vi "FB Server.vi"(0 "C2O":dbl[][](array[numeric])) -> (7 "Fx                     Fy                     Fz                    Mx                   My                    Mz":dbl[](array[numeric])=[0.39367133033328505, 0.12640519158271346, -0.035168369141984894, 0.07356448847559971, 0.08928756090020755, 0.03408632169703757])   [LabVIEW 2017]
uses:
  <vilib>/Analysis/baseanly.llb/Mean (DBL).vi
  <vilib>/Analysis/baseanly.llb/A x Vector.vi
  <vilib>/Utility/file.llb/Write To Spreadsheet File (DBL).vi
  <vilib>/Utility/file.llb/Read From Spreadsheet File (DBL).vi
  <vilib>/Analysis/NI_AALBase.lvlib
panel:
  in  "Sampling Period":dbl=30.0
  in  "Sampling Freq.":dbl=500.0
  in  "x":bool
  in  "stop":bool
  out "Waveform Chart":dynamicdata(graph)=[{"t0"=timestamp(3625740071.8186145 s since 1904-01-01), "dt"=0.002, "Y"=[1.4132434446437658, 1.4869062871436736, 1.4652020568354351, 1.4342899711432204, 1.515516408827019], "attributes"=variant("NI_ChannelName"=variant(string "Voltage_0"), "NI_UnitDescription"=variant(string "Volts"))}, {"t0"=timestamp(3625740071.8186283 s since 1904-01-01), "dt"=0.002, "Y"=[0.4493782119596065, 0.441156910799936, 0.42537201251587176, 0.4112313744050537, 0.41221793055431444], "attributes"=variant("NI_ChannelName"=variant(string "Voltage_1"), "NI_UnitDescription"=variant(string "Volts"))}, {"t0"=timestamp(3625740071.818642 s since 1904-01-01), "dt"=0.002, "Y"=[0.1241435215364698, 0.13861301307479987, 0.18070607894651378, 0.13466678811720997, 0.12841859858966923], "attributes"=variant("NI_ChannelName"=variant(string "Voltage_2"), "NI_UnitDescription"=variant(string "Volts"))}, {"t0"=timestamp(3625740071.8186564 s since 1904-01-01), "dt"=0.002, "Y"=[4.929329220143692, 4.876055168157049, 4.92110791573665, 4.952020020475538, 4.8872361419192885], "attributes"=variant("NI_ChannelName"=variant(string "Voltage_3"), "NI_UnitDescription"=variant(string "Volts"))}, {"t0"=timestamp(3625740071.8186703 s since 1904-01-01), "dt"=0.002, "Y"=[1.7019754755920375, 1.6973715480570852, 1.6858617292118738, 1.741437711535304, 1.7019754755920375], "attributes"=variant("NI_ChannelName"=variant(string "Voltage_4"), "NI_UnitDescription"=variant(string "Volts"))}, {"t0"=timestamp(3625740071.8186846 s since 1904-01-01), "dt"=0.002, "Y"=[-1.6523161496933905, -1.626994516567589, -1.6023305886073516, -1.6164712405886696, -1.6292964831977657], "attributes"=variant("NI_ChannelName"=variant(string "Voltage_5"), "NI_UnitDescription"=variant(string "Volts"))}]
  out "L2                   S                  D2                  L1                  L3                  D1":dbl[](array[numeric])=[1.4630316337186229, 0.42787128804695646, 0.14130960005293253, 1.7057243879976673, 4.913149693286444, -1.6254817957309533]
  out "Amber Check":bool[](array[boolean])
  out "Amber Check Fail":bool
  out "OMFG Check":bool[](array[boolean])
  out "OMFG Check Fail":bool
  out "Mean Convergence":dbl(graph)=0.08995560655426219
  in  "Blank Button":bool
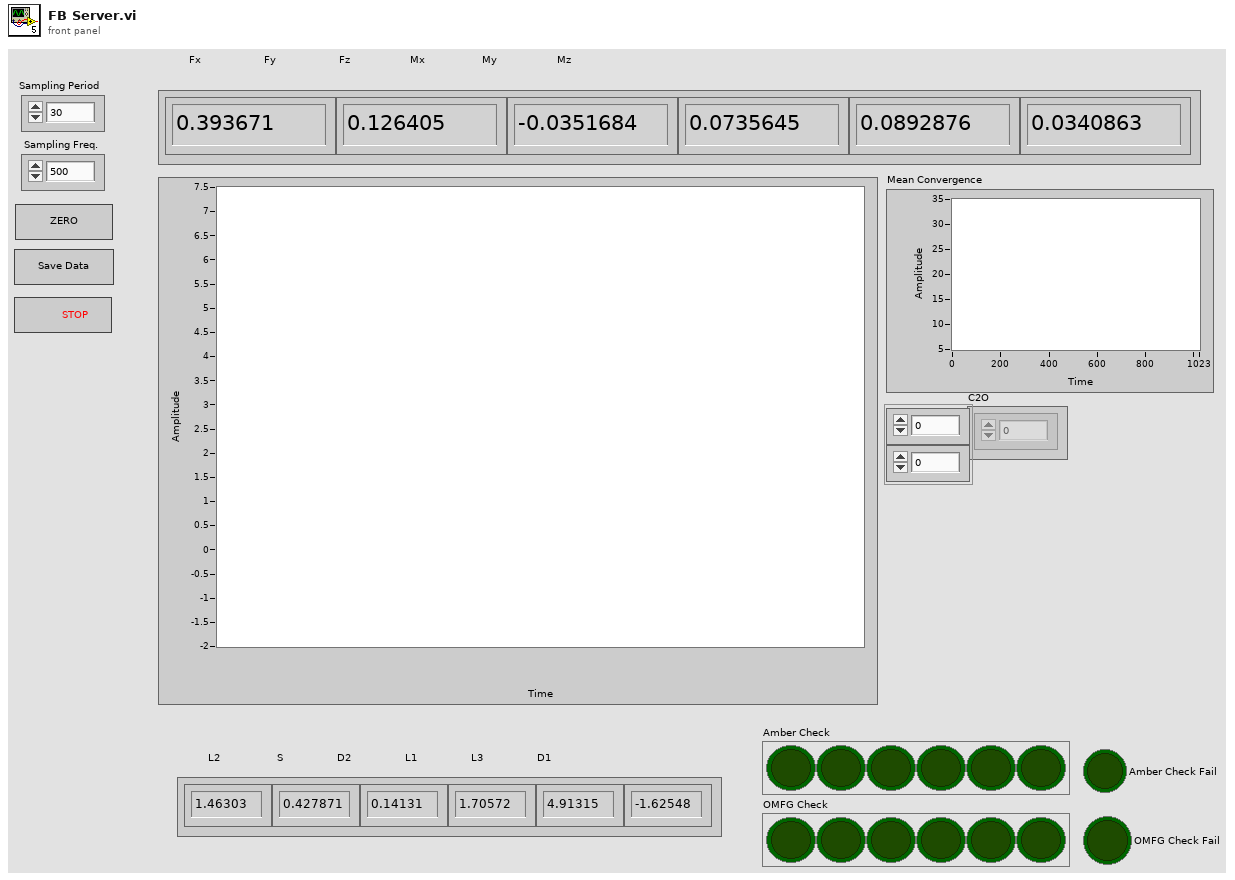
[diagram p1: front panel]
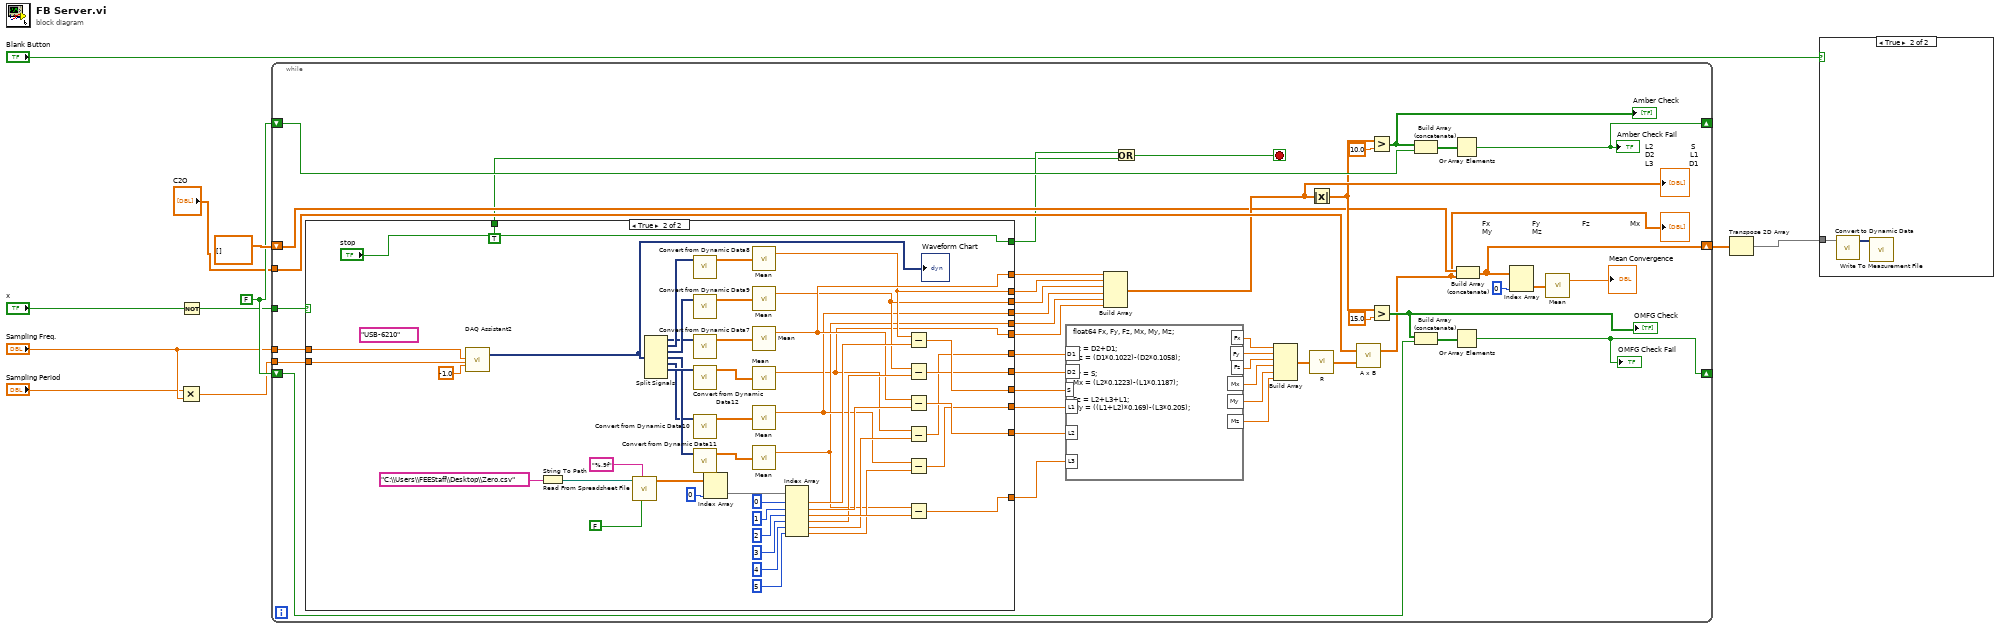
[diagram p0: block diagram]
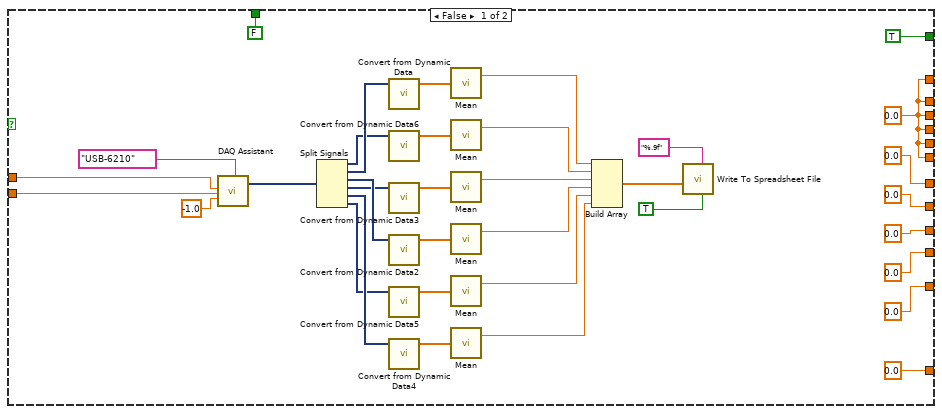
[diagram p3: hidden frame]
diagram:
  w9 = FALSE
  n1 = Multiply(x="Sampling Period", y="Sampling Freq.") -> (x*y=w7:dbl)
  n2 = Not(x="x") -> (.not. x?=w3:bool)
  n3 = while {
    tunnel: w3 -> [w56]
    tunnel: "Sampling Freq." -> [w55]
    tunnel: w7 -> [w54]
    tunnel: "C2O" -> [w53]
    shift-right: [w17] -> _
    shift-left: w9 -> [w30]
    shift-right: [w18] -> _
    shift-left: w9 -> [w25]
    shift-right: [w19] -> w11
    shift-left: dbl[][] [] -> [w20]
    stop <- w14 stop-if-true
    n4 = case shown="True" w56 {
      tunnel: [0.0 w107] -> w46
      tunnel: [0.0 w106] -> w45
      tunnel: [0.0 w125] -> w49
      tunnel: [0.0 w124] -> w48
      tunnel: [0.0 w126] -> w47
      tunnel: [0.0 w127] -> w50
      tunnel: w55 -> [w91 w140]
      tunnel: w54 -> [w90 w139]
      tunnel: [TRUE ("stop") "stop"] -> w15
      tunnel: [w58 w98] -> w38
      tunnel: [w58 w97] -> w37
      tunnel: [w58 w96] -> w36
      tunnel: [w58 w95] -> w35
      tunnel: [w58 w94] -> w34
      tunnel: [w58 w93] -> w33
      tunnel: [FALSE ("stopped") TRUE ("stopped")] -> w12
      frame False {
        w58 = 0.0
        n5 = call "DAQ Assistant"("rate"=w91, "number of samples"=w90, "timeout (s)"=-1.0, "device name"=tag "USB-6210") -> ("data"=w77:dynamicdata)  [unwired: 13 in, 2 out]
        n6 = Split Signals(w77) -> (w65:dynamicdata, w76:dynamicdata, w74:dynamicdata, w72:dynamicdata, w70:dynamicdata, w68:dynamicdata)  [unwired: 6 in]
        n7 = call "Convert from Dynamic Data"("Dynamic Data Type"=w76) -> ("Array"=w75:dbl[])  [unwired: 3 in]
        n8 = call "Convert from Dynamic Data6"("Dynamic Data Type"=w65) -> ("Array"=w61:dbl[])  [unwired: 3 in]
        n9 = call "Convert from Dynamic Data3"("Dynamic Data Type"=w72) -> ("Array"=w71:dbl[])  [unwired: 3 in]
        n10 = call "Convert from Dynamic Data2"("Dynamic Data Type"=w74) -> ("Array"=w73:dbl[])  [unwired: 3 in]
        n11 = call "Convert from Dynamic Data5"("Dynamic Data Type"=w68) -> ("Array"=w67:dbl[])  [unwired: 3 in]
        n12 = call "Convert from Dynamic Data4"("Dynamic Data Type"=w70) -> ("Array"=w69:dbl[])  [unwired: 3 in]
        n13 = call-poly <vilib>:"Mean.vi"("X"=w75) -> ("mean"=w82:dbl)  [unwired: 1 out]
        n14 = call-poly <vilib>:"Mean.vi"("X"=w61) -> ("mean"=w79:dbl)  [unwired: 1 out]
        n15 = call-poly <vilib>:"Mean.vi"("X"=w71) -> ("mean"=w62:dbl)  [unwired: 1 out]
        n16 = call-poly <vilib>:"Mean.vi"("X"=w73) -> ("mean"=w81:dbl)  [unwired: 1 out]
        n17 = call-poly <vilib>:"Mean.vi"("X"=w67) -> ("mean"=w80:dbl)  [unwired: 1 out]
        n18 = call-poly <vilib>:"Mean.vi"("X"=w69) -> ("mean"=w60:dbl)  [unwired: 1 out]
        n19 = Build Array(w82, w79, w62, w81, w80, w60) -> (w78:dbl[])
        n20 = call-poly <vilib>:"Write To Spreadsheet File.vi"("transpose? (no:F)"=TRUE, "format (%.3f)"="%.9f", "1D data"=w78) -> ()  [unwired: 5 in, 1 out]
      }
      frame True {
        (unwired) tag "USB-6210" ("device name")
        n21 = call "DAQ Assistant2"("rate"=w140, "number of samples"=w139, "timeout (s)"=-1.0) -> ("data"=w99:dynamicdata)  [unwired: 14 in, 2 out]
        "Waveform Chart" <- w99
        n22 = String To Path(string="C:\\Users\\FEEStaff\\Desktop\\Zero.csv" ("format (%.3f)")) -> (path=w108:path)
        n23 = call-poly <vilib>:"Read From Spreadsheet File.vi"("transpose (no:F)"=FALSE, "format (%.3f)"="%.9f", "file path (dialog if empty)"=w108) -> ("all rows"=w130:dbl[][])  [unwired: 4 in, 4 out]
        n24 = Split Signals(w99) -> (w115:dynamicdata, w121:dynamicdata, w119:dynamicdata, w102:dynamicdata, w101:dynamicdata, w116:dynamicdata)  [unwired: 7 in, 1 out]
        n25 = call "Convert from Dynamic Data8"("Dynamic Data Type"=w121) -> ("Array"=w120:dbl[])  [unwired: 3 in]
        n26 = call "Convert from Dynamic Data9"("Dynamic Data Type"=w119) -> ("Array"=w104:dbl[])  [unwired: 3 in]
        n27 = call "Convert from Dynamic Data7"("Dynamic Data Type"=w115) -> ("Array"=w122:dbl[])  [unwired: 3 in]
        n28 = call "Convert from Dynamic Data12"("Dynamic Data Type"=w116) -> ("Array"=w105:dbl[])  [unwired: 3 in]
        n29 = call "Convert from Dynamic Data10"("Dynamic Data Type"=w101) -> ("Array"=w118:dbl[])  [unwired: 3 in]
        n30 = call "Convert from Dynamic Data11"("Dynamic Data Type"=w102) -> ("Array"=w117:dbl[])  [unwired: 3 in]
        n31 = Index Array(array=w130, index (col)=0 ("disabled index (col)")) -> (element=w128:dbl[])  [unwired: 1 in]
        n32 = call-poly <vilib>:"Mean.vi"("X"=w120) -> ("mean"=w97:dbl)  [unwired: 1 out]
        n33 = call-poly <vilib>:"Mean.vi"("X"=w104) -> ("mean"=w96:dbl)  [unwired: 1 out]
        n34 = call-poly <vilib>:"Mean.vi"("X"=w122) -> ("mean"=w98:dbl)  [unwired: 1 out]
        n35 = call-poly <vilib>:"Mean.vi"("X"=w105) -> ("mean"=w93:dbl)  [unwired: 1 out]
        n36 = call-poly <vilib>:"Mean.vi"("X"=w118) -> ("mean"=w95:dbl)  [unwired: 1 out]
        n37 = call-poly <vilib>:"Mean.vi"("X"=w117) -> ("mean"=w94:dbl)  [unwired: 1 out]
        n38 = Index Array(array=w128, index #1=0 ("index (row)"), index #2=1 ("index (row)"), index #3=2 ("index (row)"), index #4=3 ("index (row)"), index #5=4 ("index (row)"), index #6=5 ("index (row)")) -> (element #1=w114:dbl, element #2=w113:dbl, element #3=w112:dbl, element #4=w111:dbl, element #5=w110:dbl, element #6=w103:dbl)
        n39 = Subtract(x=w97, y=w114) -> (x-y=w127:dbl)
        n40 = Subtract(x=w96, y=w111) -> (x-y=w107:dbl)
        n41 = Subtract(x=w98, y=w113) -> (x-y=w125:dbl)
        n42 = Subtract(x=w93, y=w110) -> (x-y=w106:dbl)
        n43 = Subtract(x=w95, y=w103) -> (x-y=w124:dbl)
        n44 = Subtract(x=w94, y=w112) -> (x-y=w126:dbl)
      }
    }
    n45 = formula code="float64 Fx, Fy, Fz, Mx, My, Mz;\n\nFx = D2+D1;\nMz = (D1*0.1022)-(D2*0.1058);\n\nFy = S;\nMx = (L2*0.1223)-(L1*0.1187);\n\nFz = L2+L3+L1;\nMy = ((L1+L2)*0.169)-(L3*0.205);"("D1"=w45, "D2"=w46, "S"=w50, "L1"=w48, "L2"=w49, "L3"=w47) -> ("Fx"=w44:dbl, "Fy"=w43:dbl, "Fz"=w42:dbl, "Mx"=w41:dbl, "My"=w40:dbl, "Mz"=w39:dbl)
    n46 = Build Array(w38, w37, w36, w35, w34, w33) -> (w32:dbl[])
    "L2                   S                  D2                  L1                  L3                  D1" <- w32
    n47 = Or(x=w15, y=w12) -> (x .or. y?=w14:bool)
    n48 = Build Array(w44, w43, w42, w41, w40, w39) -> (w51:dbl[])
    n49 = Absolute Value(x=w32) -> (abs(x)=w27:dbl[])
    n50 = call "R.vi"("1x6"=w51) -> ("27x1"=w52:dbl[])
    n51 = call-poly <vilib>:"A x B.vi"("Vector"=w52, "A"=w53) -> ("A x Vector"=w16:dbl[])  [unwired: 1 out]
    "Fx                     Fy                     Fz                    Mx                   My                    Mz" <- w16
    n52 = Greater?(x=w27, y=10.0 ("Numeric")) -> (0:w28:bool[])
    "Amber Check" <- w28
    n53 = Greater?(x=w27, y=15.0) -> (0:w23:bool[])
    "OMFG Check" <- w23
    n54 = Build Array (concatenate)(w28, w30) -> (w29:bool[])
    n55 = Build Array (concatenate)(w23, w25) -> (w24:bool[])
    n56 = Or Array Elements(Boolean array=w29) -> (logical OR=w17:bool)
    "Amber Check Fail" <- w17
    n57 = Or Array Elements(Boolean array=w24) -> (logical OR=w18:bool)
    "OMFG Check Fail" <- w18
    n58 = Build Array (concatenate)(w20, w16) -> (w19:dbl[][])
    n59 = Index Array(array=w19, index (col)=0 ("index")) -> (element=w21:dbl[])  [unwired: 1 in]
    n60 = call-poly <vilib>:"Mean.vi"("X"=w21) -> ("mean"=→"Mean Convergence":dbl)  [unwired: 1 out]
  }
  n61 = Transpose 2D Array(2D array=w11) -> (transposed array=w2:dbl[][])
  n62 = case shown="True" "Blank Button" {
    tunnel: w2 -> [_ w142]
    frame False {
    }
    frame True {
      n63 = call "Convert to Dynamic Data"("2D Array"=w142) -> ("Dynamic Data Type"=w141:dynamicdata)  [unwired: 3 in]
      n64 = call "Write To Measurement File"("Signals"=w141) -> ()  [unwired: 16 in, 3 out]
    }
  }
